vi "Version Compare.vi"(2 "Consider Date? (f)":bool, 3 "Version 1":T1 {"Build Date/Time" format="%<%X\n%x>T"}, 4 "Version 2":T1 {"Build Date/Time" format="%<%X\n%x>T"}) -> (0 "Version Comparison":T2(ring), 1 "Newest Version":T1 {"Build Date/Time" format="%<%X\n%x>T"})   [LabVIEW 2011]
uses:
  OGAB Version.ctl
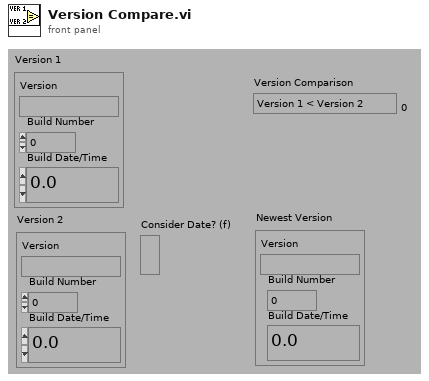
[diagram p1: front panel]
types:
  T1 = typedef "OGAB Version.ctl" = cluster{"Version":string, "Build Number":u32, "Build Date/Time":dbl}
  T2 = enum16{"Version 1 < Version 2", "Version 1 = Version 2", "Version 1 > Version 2"}
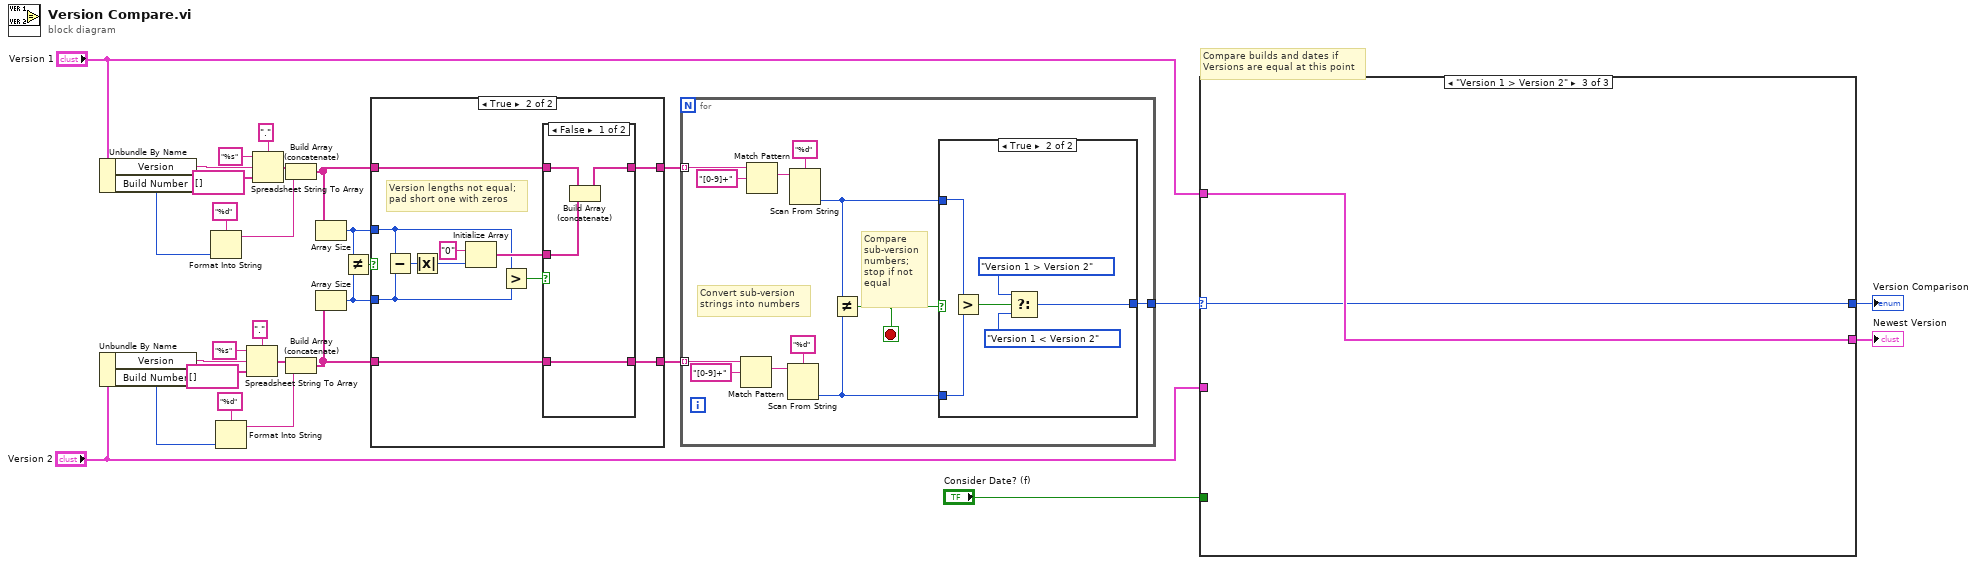
[diagram p0: block diagram]
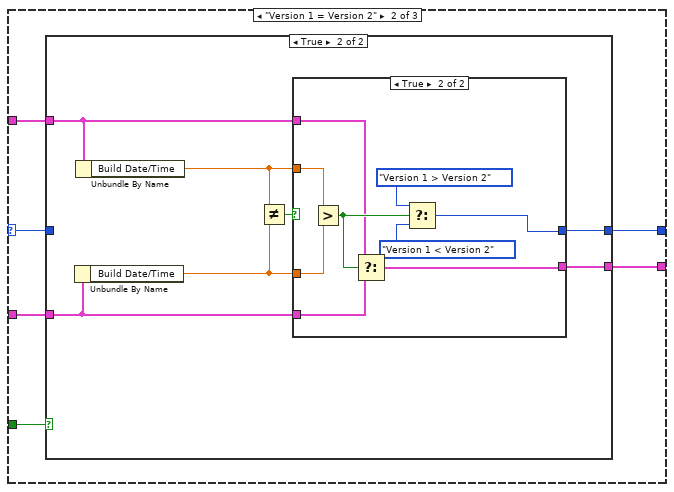
[diagram p3: hidden frame]
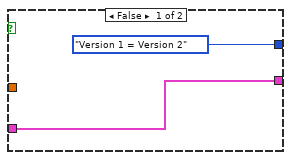
[diagram p5: hidden frame]
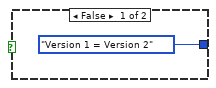
[diagram p6: hidden frame]
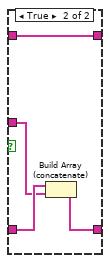
[diagram p8: hidden frame]
diagram:
  # "Compare builds and dates if\nVersions are equal at this point"
  n1 = Unbundle By Name("Version 1") -> ("Version"=w27:string, "Build Number"=w5:u32)
  n2 = Unbundle By Name("Version 2") -> ("Version"=w22:string, "Build Number"=w6:u32)
  n3 = Format Into String(format string="%d", w5) -> (resulting string=w3:string)  [unwired: 2 in, 1 out]
  n4 = Format Into String(format string="%d", w6) -> (resulting string=w1:string)  [unwired: 2 in, 1 out]
  n5 = Spreadsheet String To Array(delimiter (Tab)=".", format string="%s", spreadsheet string=w22, array type (2D Dbl)=string[] []) -> (array=w19:string[])
  n6 = Spreadsheet String To Array(delimiter (Tab)=".", format string="%s", spreadsheet string=w27, array type (2D Dbl)=string[] []) -> (array=w20:string[])
  n7 = Build Array (concatenate)(w20, w3) -> (w4:string[])
  n8 = Build Array (concatenate)(w19, w1) -> (w2:string[])
  n9 = Array Size(array=w4) -> (size(s)=w18:i32)
  n10 = Array Size(array=w2) -> (size(s)=w17:i32)
  n11 = Not Equal?(x=w18, y=w17) -> (x != y?=w21:bool)
  n12 = case shown="True" w21 {
    tunnel: [w31 w32] -> w16
    tunnel: w4 -> [w31 w33]
    tunnel: [w30 w38] -> w15
    tunnel: w2 -> [w30 w40]
    tunnel: w18 -> [_ w36]
    tunnel: w17 -> [_ w35]
    frame False {
      # "Version lengths are equal"
    }
    frame True {
      # "Version lengths not equal;\npad short one with zeros"
      n13 = Subtract(x=w36, y=w35) -> (x-y=w41:i32)
      n14 = Absolute Value(x=w41) -> (abs(x)=w37:i32)
      n15 = Initialize Array("0" ("format string"), w37) -> (w39:string[])
      n16 = Greater?(x=w36, y=w35) -> (0:w34:bool)
      n17 = case shown="False" w34 {
        tunnel: w40 -> [w43 w50]
        tunnel: w39 -> [w45 w49]
        tunnel: [w43 w48] -> w38
        tunnel: w33 -> [w46 w47]
        tunnel: [w44 w47] -> w32
        frame False {
          n18 = Build Array (concatenate)(w46, w45) -> (w44:string[])
        }
        frame True {
          n19 = Build Array (concatenate)(w50, w49) -> (w48:string[])
        }
      }
    }
  }
  n20 = for {
    tunnel: w16 -> [w62] mode=indexing
    tunnel: w15 -> [w59] mode=indexing
    tunnel: [w51] -> w14
    stop <- w54 stop-if-true
    # "Compare\nsub-version\nnumbers;\nstop if not\nequal"
    # "Convert sub-version\nstrings into numbers"
    n21 = Match Pattern(string=w59, regular expression="[0-9]+") -> (match substring=w55:string)  [unwired: 4 out]
    n22 = Match Pattern(string=w62, regular expression="[0-9]+") -> (match substring=w57:string)  [unwired: 4 out]
    n23 = Scan From String(format string="%d", input string=w55) -> (output 1=w52:i32)  [unwired: 2 in, 4 out]
    n24 = Scan From String(format string="%d", input string=w57) -> (output 1=w53:i32)  [unwired: 2 in, 4 out]
    n25 = Not Equal?(x=w53, y=w52) -> (x != y?=w54:bool)
    n26 = case shown="True" w54 {
      tunnel: w53 -> [_ w69]
      tunnel: w52 -> [_ w68]
      tunnel: [T2."Version 1 = Version 2" ("Version Comparison") w64] -> w51
      frame False {
      }
      frame True {
        n27 = Greater?(x=w69, y=w68) -> (0:w67:bool)
        n28 = Select(t=T2."Version 1 > Version 2" ("Version Comparison"), s=w67, f=T2."Version 1 < Version 2" ("Version Comparison")) -> (s? t:f=w64:T2)
      }
    }
  }
  n29 = case shown="\"Version 1 > Version 2\"" w14 {
    selector: w14 -> [w71 w72 w98]
    tunnel: "Version 1" -> [_ w76 w99]
    tunnel: "Version 2" -> [w70 w75 _]
    tunnel: [w71 w77 w98] -> w11
    tunnel: [w70 w74 w99] -> w10
    tunnel: "Consider Date? (f)" -> [_ w73 _]
    frame "Version 1 < Version 2", Default {
    }
    frame "Version 1 = Version 2" {
      n30 = case shown="True" w73 {
        tunnel: [w79 w86] -> w77
        tunnel: w76 -> [_ w85]
        tunnel: w75 -> [w78 w84]
        tunnel: [w78 w83] -> w74
        tunnel: w72 -> [w79 _]
        frame False {
        }
        frame True {
          n31 = Unbundle By Name(w84) -> ("Build Date/Time"=w81:dbl)
          n32 = Unbundle By Name(w85) -> ("Build Date/Time"=w82:dbl)
          n33 = Not Equal?(x=w82, y=w81) -> (x != y?=w80:bool)
          n34 = case shown="True" w80 {
            tunnel: w85 -> [_ w92]
            tunnel: w84 -> [w88 w91]
            tunnel: [w88 w90] -> w83
            tunnel: [T2."Version 1 = Version 2" ("Version Comparison") w89] -> w86
            tunnel: w82 -> [_ w94]
            tunnel: w81 -> [_ w93]
            frame False {
            }
            frame True {
              n35 = Greater?(x=w94, y=w93) -> (0:w95:bool)
              n36 = Select(t=w92, s=w95, f=w91) -> (s? t:f=w90:T1)
              n37 = Select(t=T2."Version 1 > Version 2" ("Version Comparison"), s=w95, f=T2."Version 1 < Version 2" ("Version Comparison")) -> (s? t:f=w89:T2)
            }
          }
        }
      }
    }
    frame "Version 1 > Version 2" {
    }
  }
  "Version Comparison" <- w11
  "Newest Version" <- w10
